vi "SalvaImpostazioniFunzioniCorrettrici_INPUT.vi"(11 "Valore letto da DAQ":dbl) -> ()   [LabVIEW 2019]
uses:
  <vilib>/Utility/miscctls.llb/LVRowAndColumnTypeDef.ctl
  <vilib>/Analysis/6fits.llb/Curve Fitting Criteria.ctl
  <vilib>/Analysis/polynomials.llb/Polynomial Plot (Range).vi
  <vilib>/Analysis/NI_AALPro.lvlib
panel:
  out "Sensore selezionato":string
  in  "Elimina Funzione Correttrice":bool
  out "Ingresso Selezionato":string
  in  "Ordine Polinomio Fit":i32=2
  out "Contenuto file":string[][](array[string])
  out "Indice Sensore":i32
  in  "Tabella Acquisizioni":i32(listbox)
  in  "Valore Letto da sensore":dbl
  in  "Acquisici Punto":bool
  in  "Salva Dati":bool
  in  "Analizza Dati":bool
  in  "Elimina Ultimo Punto":bool
  in  "stop":bool
  out "Graph":cluster{"Ramp Pattern":dbl[], "P(A)":dbl[]}[](graph)
  in  "Stato Sensori":i32(listbox)
  out "transposed array":string[][](array[string])
  out "Array":string[][](array[string])
  out "array w/ subset deleted":string[][](array[string])
  out "output array 2":string[][](array[string])
  out "output array":string[][](array[string])
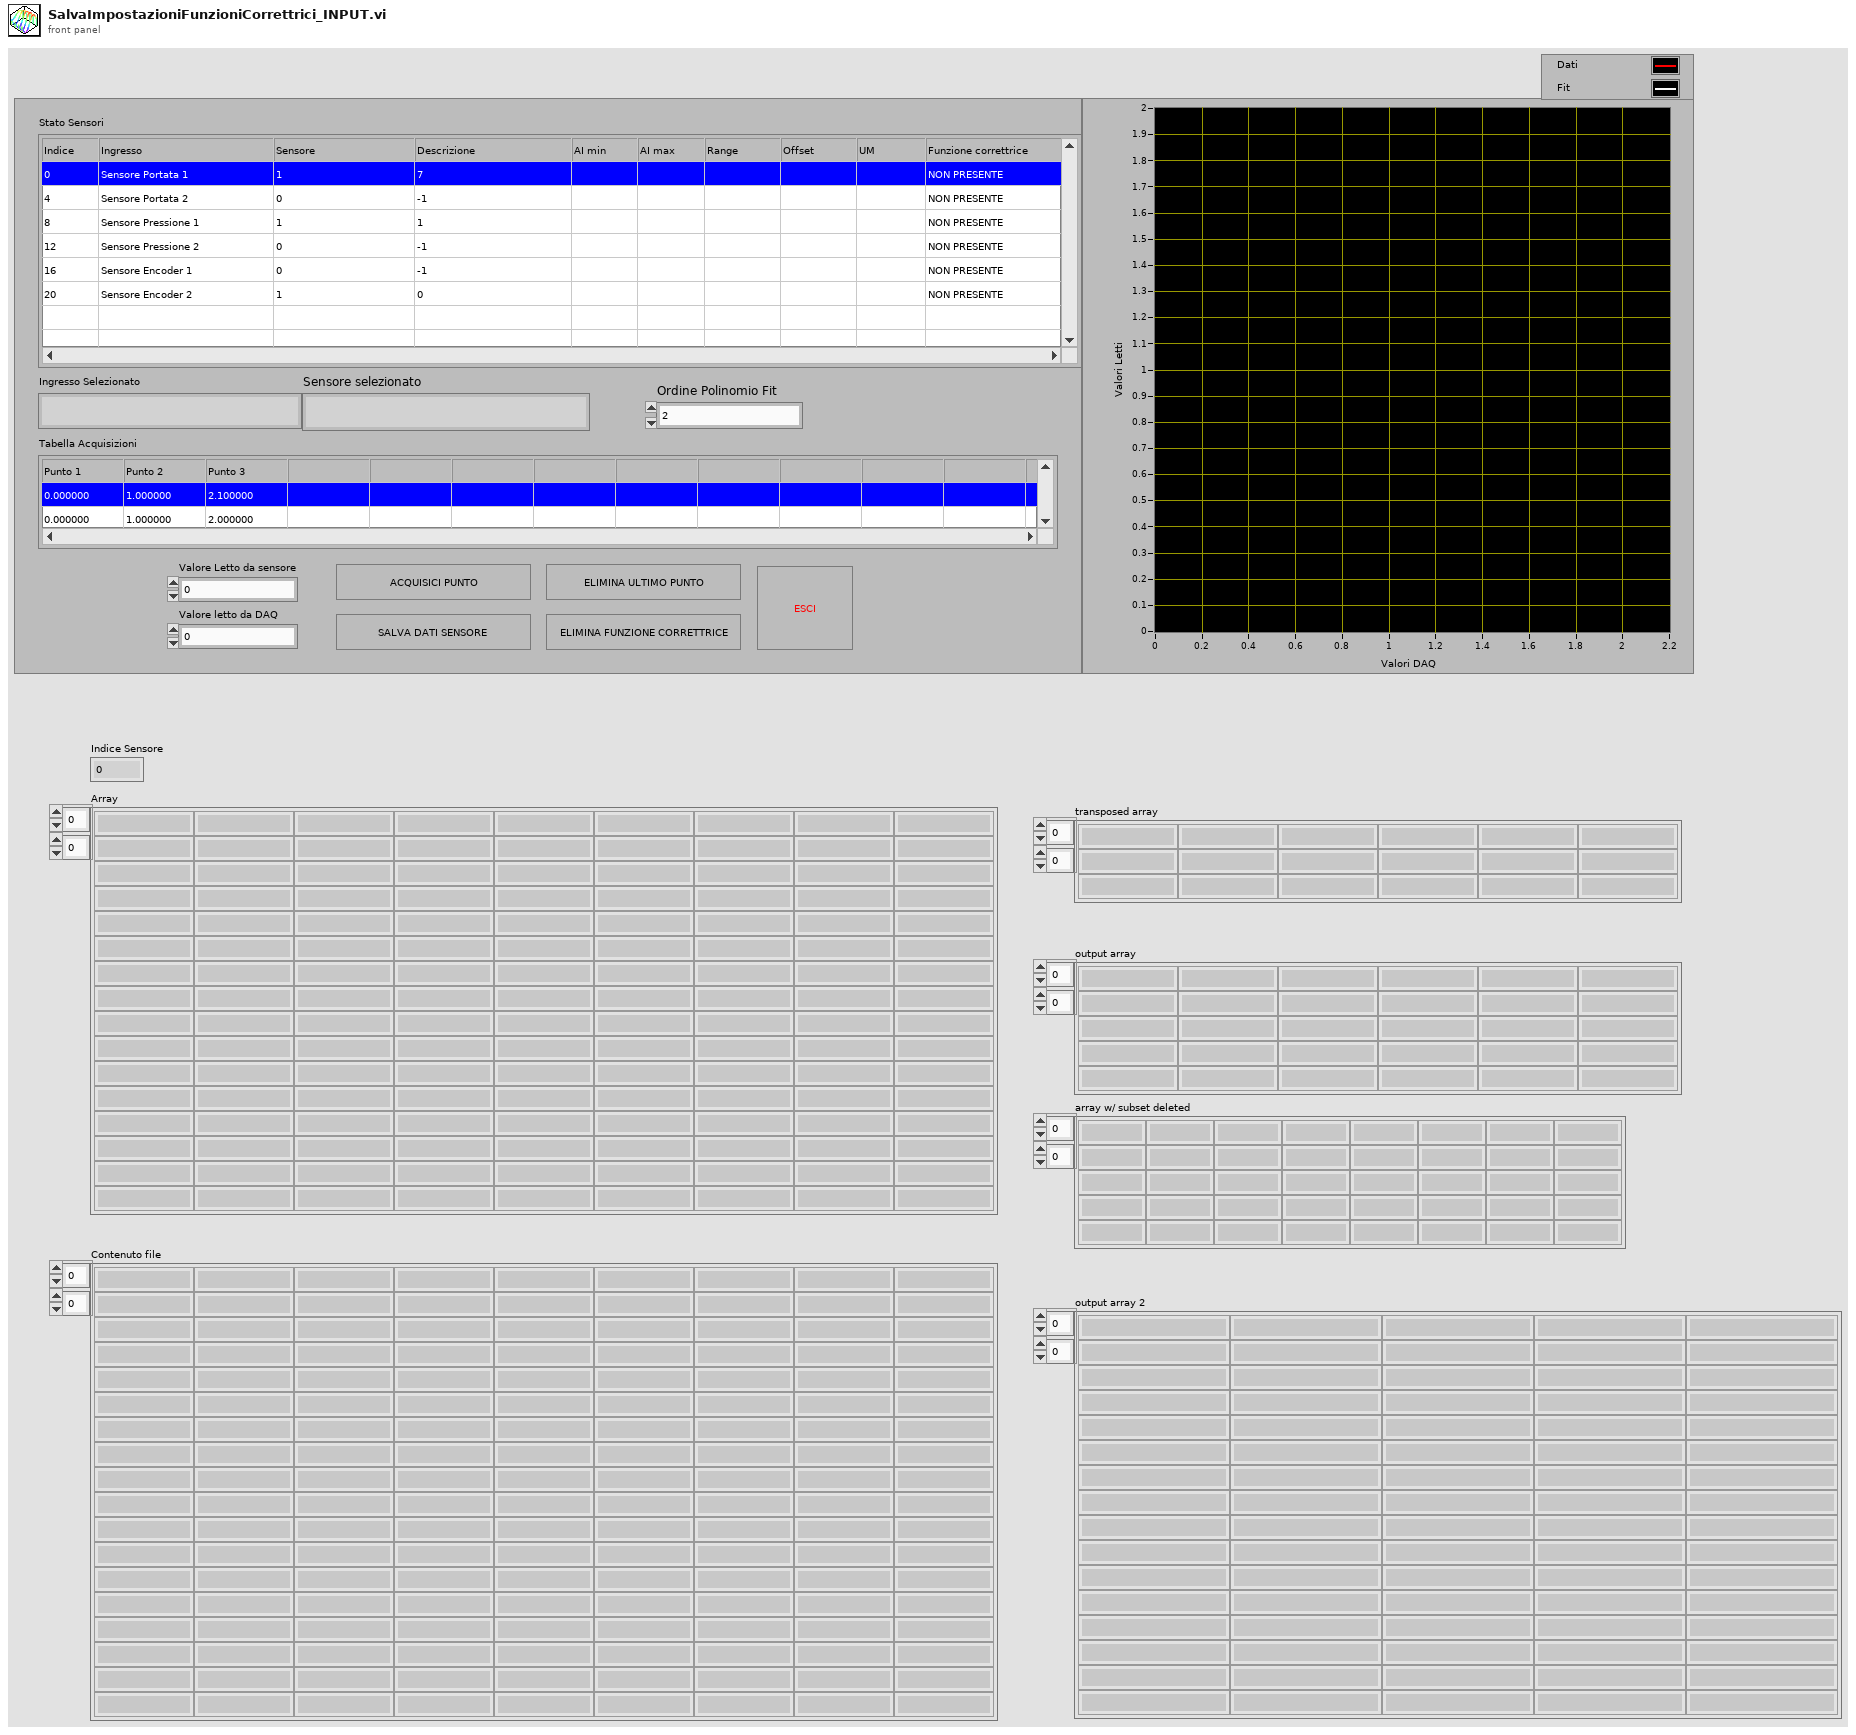
[diagram p1: front panel]
types:
  T1 = typedef "LVRowAndColumnTypeDef.ctl" = cluster{"Row":i32, "Column":i32}
  T2 = enum16{"open", "replace", "create", "open or create", "replace or create", "replace or create with confirmation"}
  T3 = typedef "NI_AALPro.lvlib/Curve Fitting Criteria.ctl" = u16
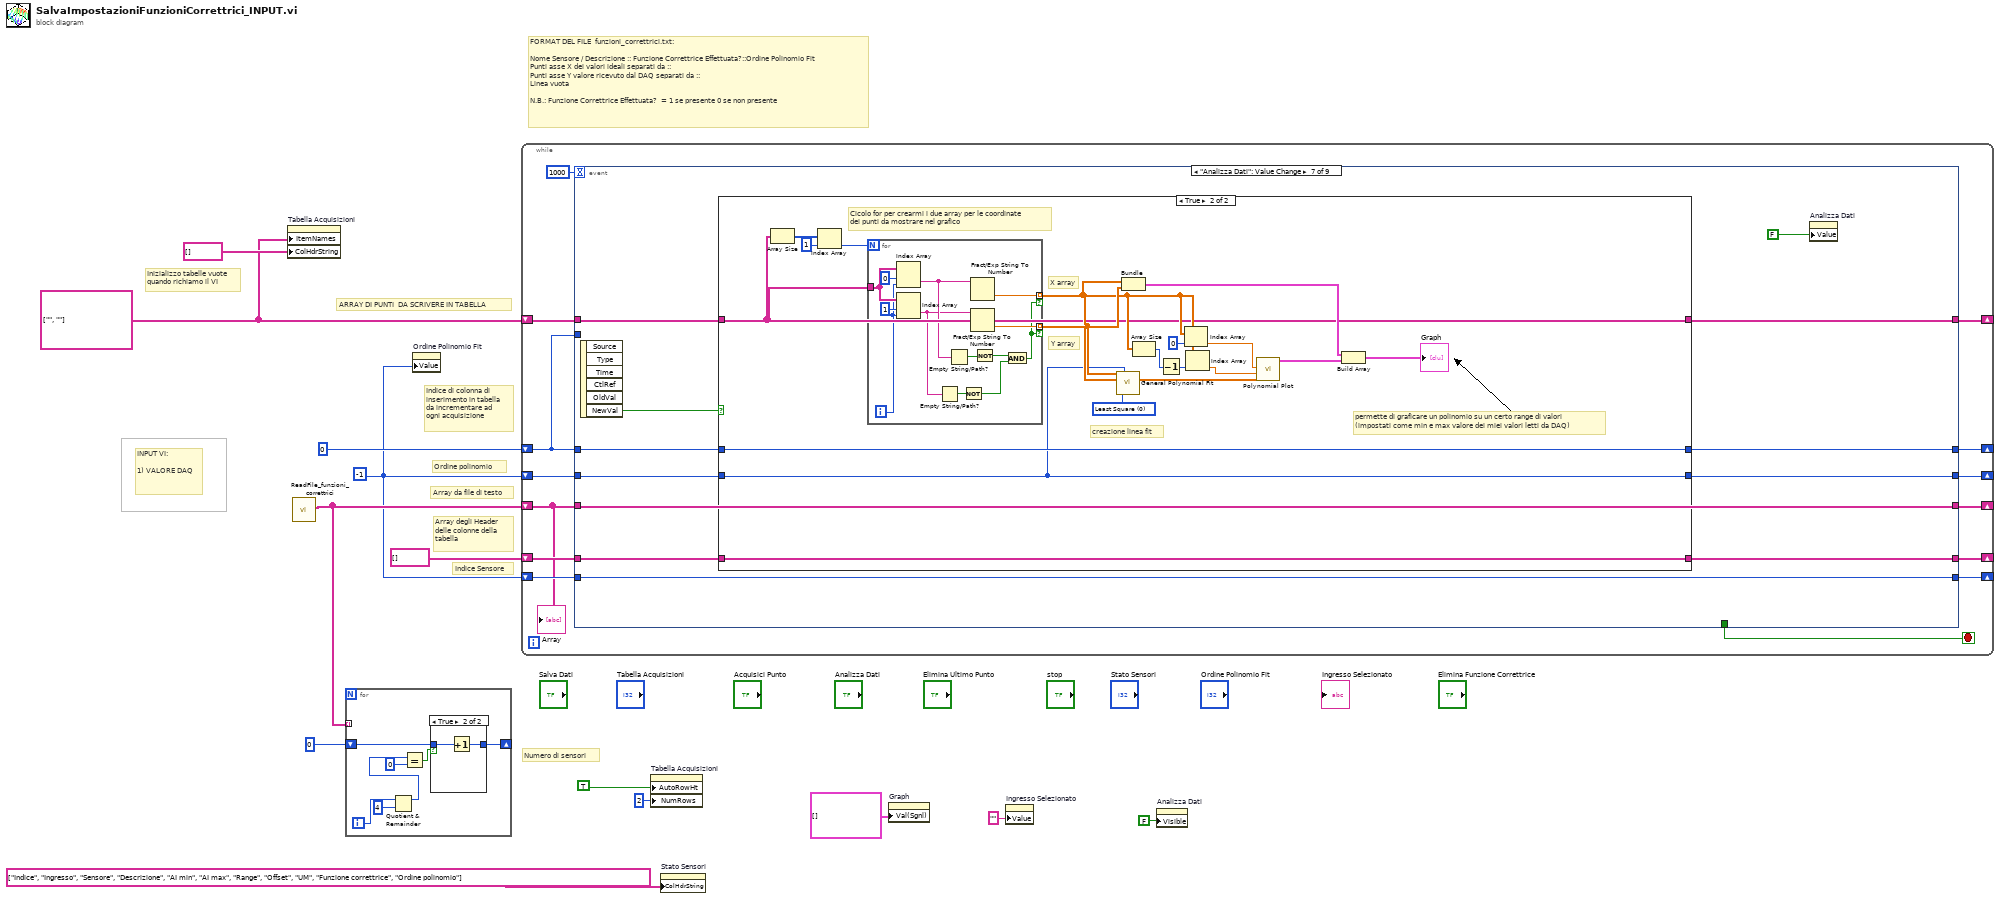
[diagram p0: block diagram]
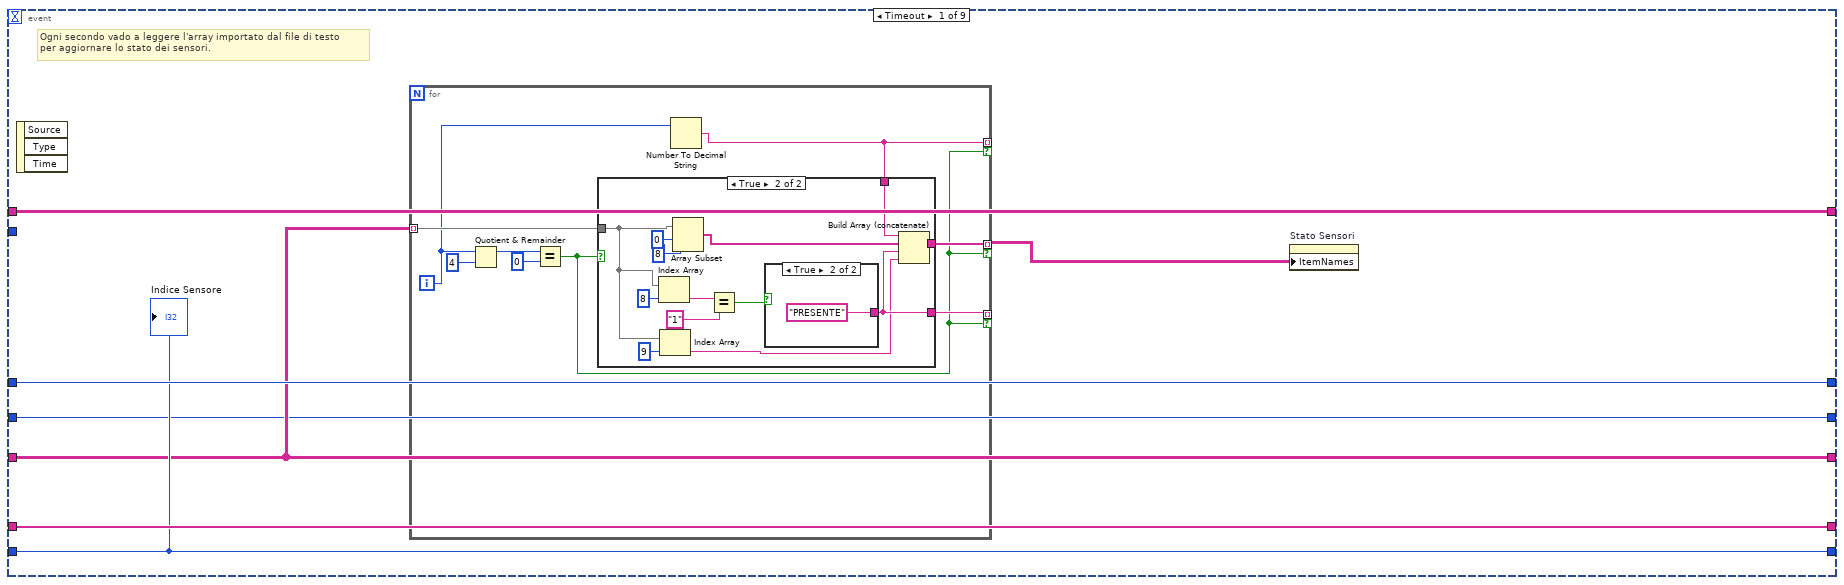
[diagram p3: hidden frame]
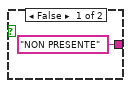
[diagram p5: hidden frame]
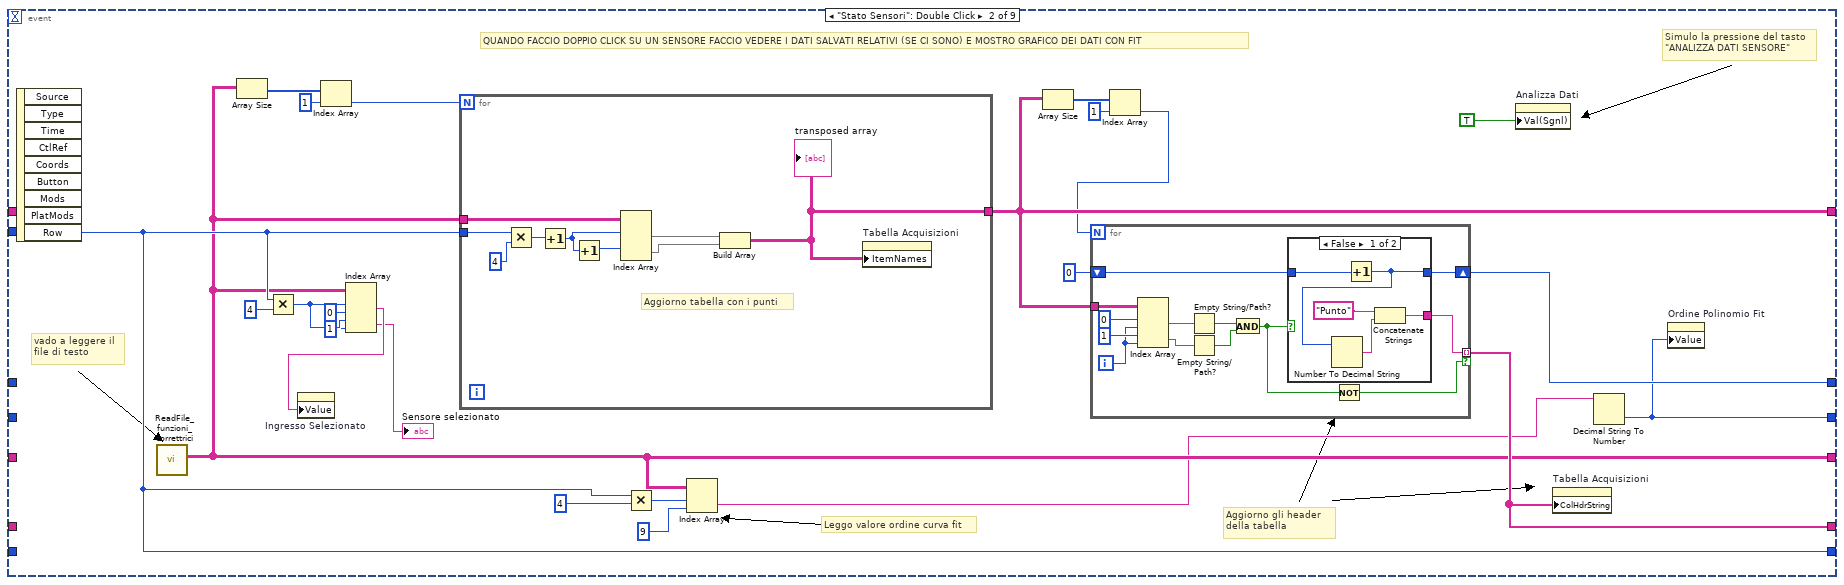
[diagram p6: hidden frame]
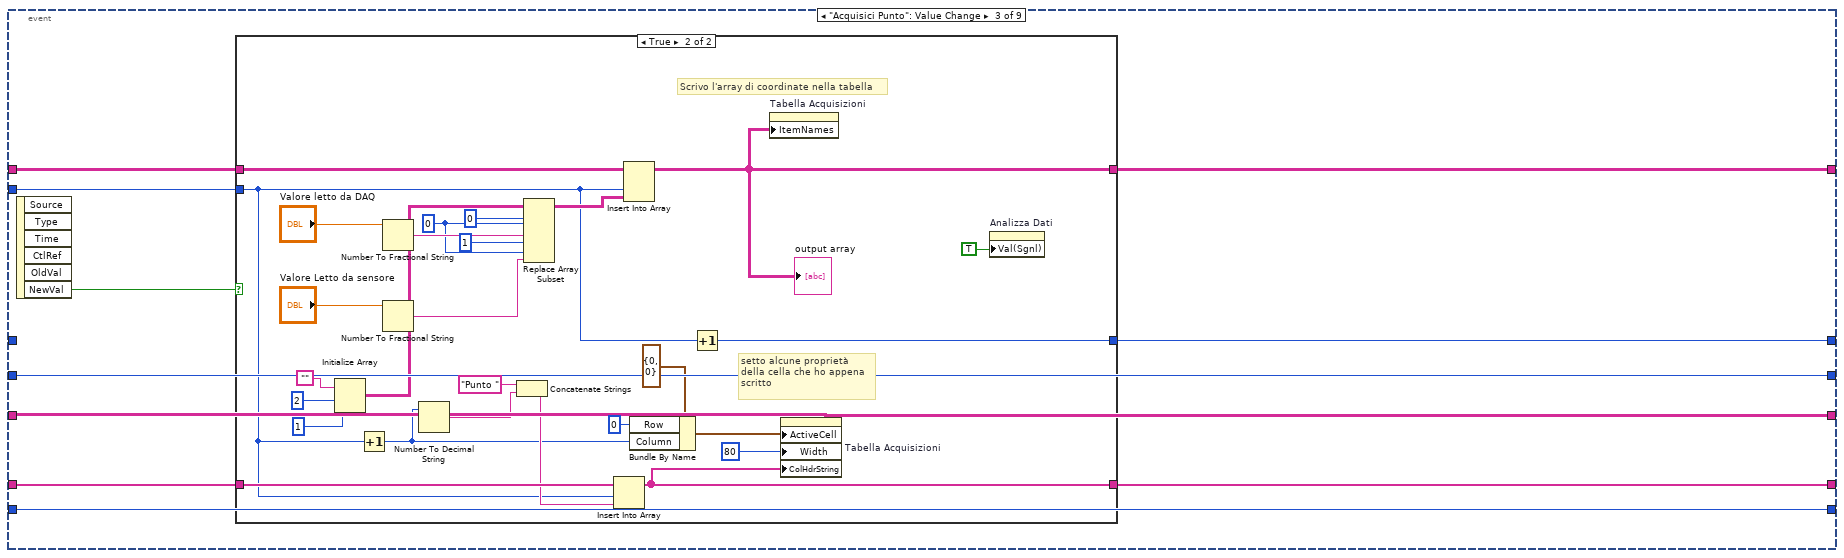
[diagram p8: hidden frame]
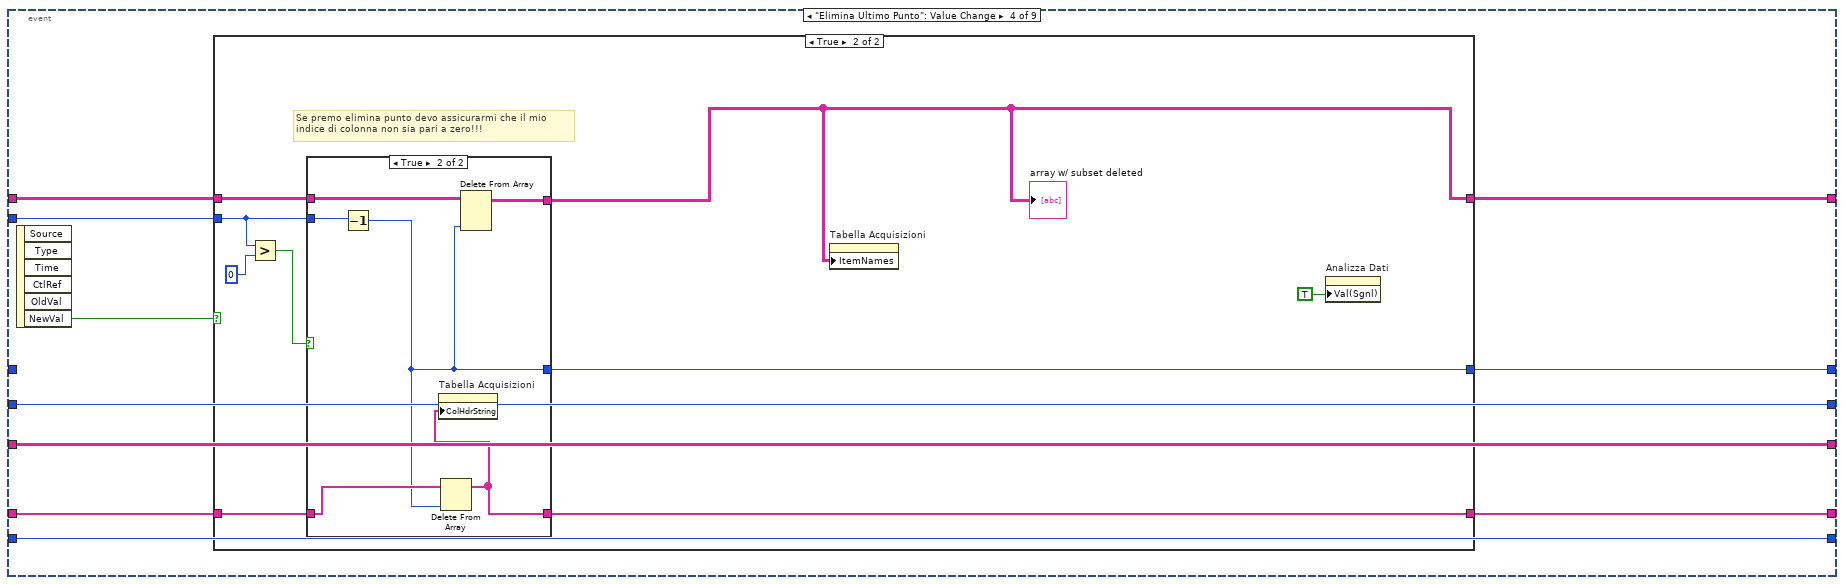
[diagram p10: hidden frame]
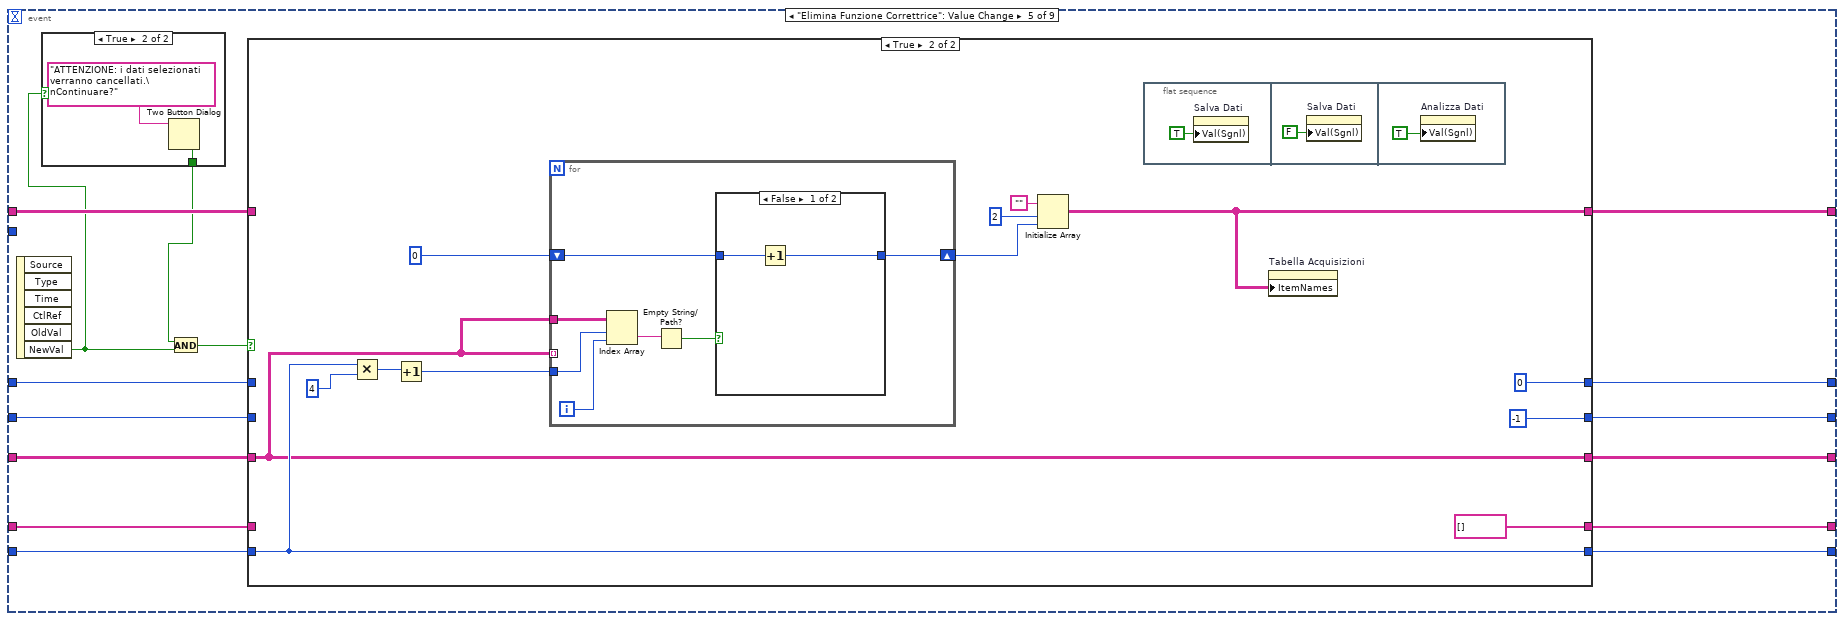
[diagram p13: hidden frame]
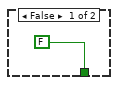
[diagram p14: hidden frame]
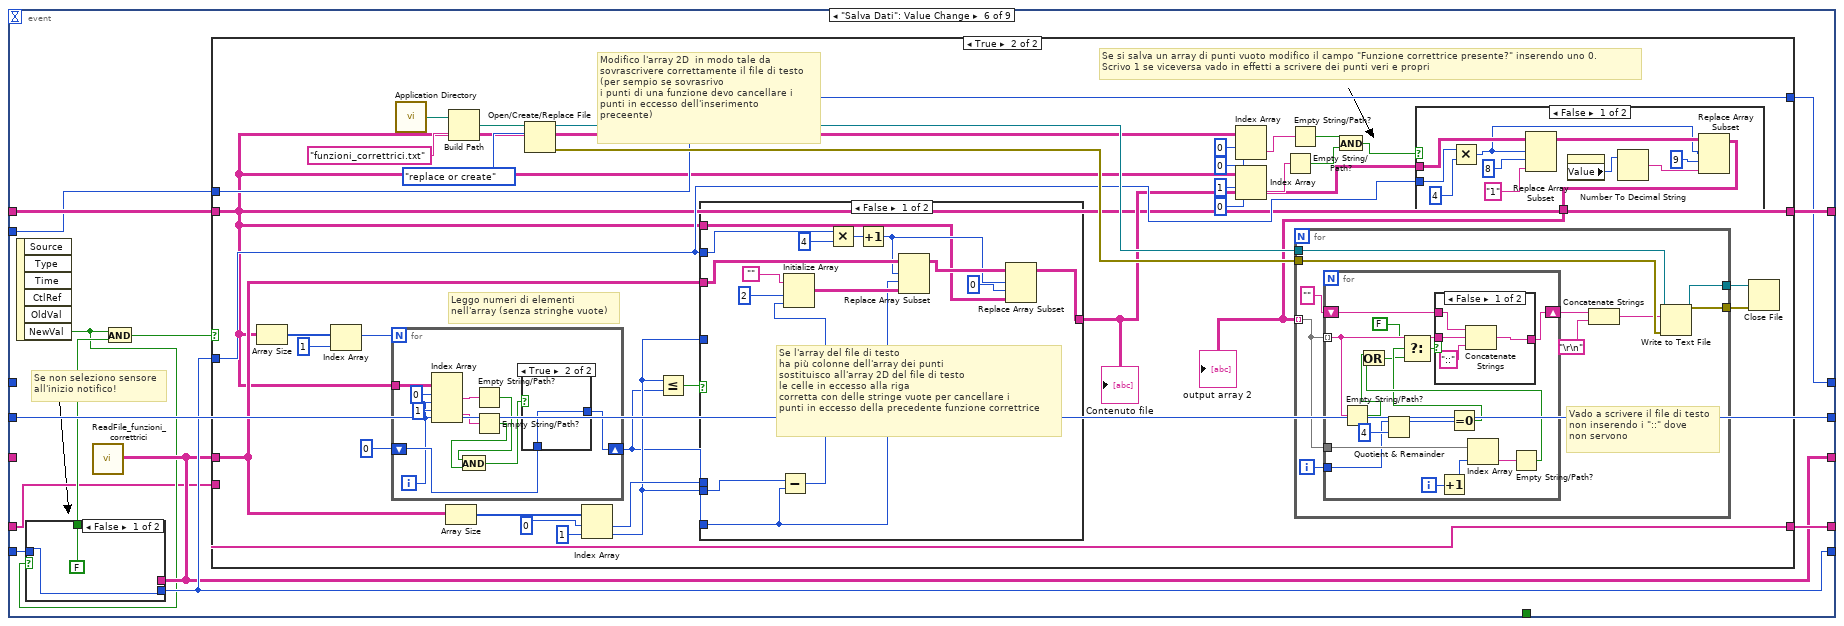
[diagram p17: hidden frame]
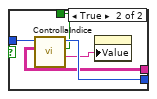
[diagram p18: hidden frame]
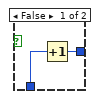
[diagram p20: hidden frame]
diagram:
  w2 = -1 ("Value")
  w6 = string[][] [[""], [""]] ("Item Names")
  # "FORMAT DEL FILE  funzioni_correttrici.txt:\n\nNome Sensore / Descrizione :: Funzione Correttrice Effettuata?::Ordine Polinomio Fit \nPunti asse X dei valori ideali separati da ::\nPunti asse Y valore ricevuto dal DAQ separati da ::\nLinea vuota\n\nN.B.: Funzione Correttrice Effettuata?  = 1 se presente 0 se non presente"
  # "Ordine polinomio"
  # "Numero di sensori"
  # "INPUT VI:\n\n1) VALORE DAQ"
  # "Array da file di testo"
  # "Indice Sensore"
  # "Array degli Header\ndelle colonne della \ntabella"
  # "Indice di colonna di \ninserimento in tabella\nda incrementare ad \nogni acquisizione"
  # "ARRAY DI PUNTI  DA SCRIVERE IN TABELLA"
  # "Inizializzo tabelle vuote\nquando richiamo il VI"
  n1 = property on="Tabella Acquisizioni" class="MCListbox (strict)"("ItemNames"=w6, "ColHdrString"=string[] [] ("Column Header Strings[]")) -> ()  [unwired: 2 in, 2 out]
  n2 = call "ReadFile_funzioni_correttrici.vi"() -> ("Contenuto file"=w4:string[][])  [unwired: 11 in]
  n3 = for {
    tunnel: w4 -> [_] mode=indexing
    shift-right: [w17] -> _
    shift-left: 0 -> [w18]
    i -> [w20]
    n4 = Quotient & Remainder(x=w20, y=4) -> (x-y*floor(x/y)=w16:i32)  [unwired: 1 out]
    n5 = Equal?(x=w16, y=0) -> (x = y?=w14:bool)
    n6 = case shown="True" w14 {
      tunnel: w18 -> [w21 w23]
      tunnel: [w21 w22] -> w17
      frame False {
      }
      frame True {
        n7 = Increment(x=w23) -> (x+1=w22:i32)
      }
    }
  }
  n8 = property on="Ordine Polinomio Fit" class="DigNum (strict)"("Value"=w2) -> ()  [unwired: 2 in, 2 out]
  n9 = while {
    shift-right: [w36] -> _
    shift-left: 0 -> [w30]
    shift-right: [w35] -> _
    shift-left: w6 -> [w37]
    shift-right: [w33] -> _
    shift-left: string[] [] ("Column Header Strings[]") -> [w34]
    shift-right: [w29] -> _
    shift-left: w4 -> [w26]
    shift-right: [w27] -> _
    shift-left: w2 -> [w32]
    shift-right: [w25] -> _
    shift-left: w2 -> [w24]
    stop <- w31 stop-if-true
    n10 = event shown="[6] \"Analizza Dati\": Value Change" {
      selector: _ -> [_ _ _ _ _ _ _ _ _]
      dyn-events: _ -> [_ _ _ _ _ _ _ _ _]
      timeout: 1000 -> [_ _ _ _ _ _ _ _ _]
      tunnel: w37 -> [w44 _ w129 w169 w202 w253 w410 w454 _]
      tunnel: w30 -> [_ _ w128 w168 _ w250 _ _ _]
      tunnel: [w43 w84 w127 w166 w198 w251 w409 w450 _] -> w36
      tunnel: [w44 w89 w126 w167 w201 w252 w411 w454 _] -> w35
      tunnel: w34 -> [w42 _ w125 w164 w195 w242 w407 w453 _]
      tunnel: [w42 w83 w124 w165 w196 w254 w406 w453 _] -> w33
      tunnel: w26 -> [w40 _ w123 w163 w205 _ w405 w452 _]
      tunnel: w32 -> [w41 _ w122 w162 w204 w248 w404 w451 _]
      tunnel: [_ _ _ _ _ _ _ _ TRUE] -> w31
      tunnel: w30 -> [w43 _ _ _ w197 _ w408 w450 _]
      tunnel: [w40 w73 w123 w163 w206 w244 w405 w452 _] -> w29
      tunnel: [w41 w74 w122 w162 w203 w247 w404 w451 _] -> w27
      tunnel: [w39 w78 w121 w161 w199 w249 w402 w449 _] -> w25
      tunnel: w24 -> [w39 _ w121 w161 w200 w249 w401 _ _]
      event Timeout {
        # "Ogni secondo vado a leggere l'array importato dal file di testo \nper aggiornare lo stato dei sensori."
        n11 = event-data() -> ()  [unwired: 1 in, 3 out]
        n12 = for {
          tunnel: w40 -> [w50] mode=indexing
          tunnel: [w49] -> _ mode=indexing if=w47
          tunnel: [w48] -> w38 mode=indexing if=w47
          tunnel: [w45] -> _ mode=indexing if=w47
          i -> [w46]
          n13 = Quotient & Remainder(x=w46, y=4) -> (x-y*floor(x/y)=w52:i32)  [unwired: 1 out]
          n14 = Equal?(x=w52, y=0) -> (x = y?=w47:bool)
          n15 = Number To Decimal String(number=w46) -> (decimal integer string=w45:string)  [unwired: 1 in]
          n16 = case shown="True" w47 {
            tunnel: w50 -> [_ w56]
            tunnel: [_ w59] -> w48
            tunnel: [_ w57] -> w49
            tunnel: w45 -> [_ w58]
            frame False {
            }
            frame True {
              n17 = Index Array(array=w56, index=8) -> (element=w65:string)
              n18 = Index Array(array=w56, index=9) -> (element=w54:string)
              n19 = Array Subset(array=w56, index=0, length=8) -> (w62:string[])
              n20 = Equal?(x=w65, y="1") -> (x = y?=w63:bool)
              n21 = case shown="True" w63 {
                tunnel: ["NON PRESENTE" "PRESENTE"] -> w57
                frame False {
                }
                frame True {
                }
              }
              n22 = Build Array (concatenate)(w58, w62, w57, w54) -> (w59:string[])
            }
          }
        }
        n23 = property on="Stato Sensori" class="MCListbox (strict)"("ItemNames"=w38) -> ()  [unwired: 2 in, 2 out]
        "Indice Sensore" <- w41
      }
      event "Stato Sensori": Double Click {
        # "Leggo valore ordine curva fit"
        # "Aggiorno gli header \ndella tabella"
        # "Simulo la pressione del tasto\n\"ANALIZZA DATI SENSORE\""
        # "QUANDO FACCIO DOPPIO CLICK SU UN SENSORE FACCIO VEDERE I DATI SALVATI RELATIVI (SE CI SONO) E MOSTRO GRAFICO DEI DATI CON FIT"
        # "vado a leggere il \nfile di testo"
        n24 = event-data() -> ("Row"=w74:i32)  [unwired: 1 in, 8 out]
        n25 = call "ReadFile_funzioni_correttrici.vi"() -> ("Contenuto file"=w73:string[][])  [unwired: 11 in]
        n26 = Array Size(array=w73) -> (size(s)=w91:i32[])
        n27 = Multiply(x=w74, y=4) -> (x*y=w72:i32)
        n28 = Index Array(array=w91, index=1) -> (element=w92:i32)
        n29 = Index Array(array=w73, index (row) #1=w72, index (col) #1=0 ("disabled index (col)"), index (row) #2=w72, index (col) #2=1 ("disabled index (col)")) -> (element #1=w76:string, element #2=→"Sensore selezionato":string)
        n30 = property on="Ingresso Selezionato" class="Str"("Value"=w76) -> ()  [unwired: 2 in, 2 out]
        n31 = for {
          N: w92 -> [_]
          tunnel: w73 -> [w120]
          tunnel: w74 -> [w119]
          tunnel: [w112] -> w89
          # "Aggiorno tabella con i punti"
          n32 = Multiply(x=w119, y=4) -> (x*y=w117:i32)
          n33 = Increment(x=w117) -> (x+1=w115:i32)
          n34 = Increment(x=w115) -> (x+1=w116:i32)
          n35 = Index Array(array=w120, index (row) #1=w115, index (row) #2=w116) -> (element #1=w114:string[], element #2=w113:string[])  [unwired: 2 in]
          n36 = Build Array(w114, w113) -> (w112:string[][])
          "transposed array" <- w112
          n37 = property on="Tabella Acquisizioni" class="MCListbox (strict)"("ItemNames"=w112) -> ()  [unwired: 2 in, 2 out]
        }
        n38 = Multiply(x=w74, y=4) -> (x*y=w81:i32)
        n39 = Index Array(array=w73, index (row)=w81, index (col)=9 ("disabled index (col)")) -> (element=w69:string)
        n40 = Array Size(array=w89) -> (size(s)=w88:i32[])
        n41 = Index Array(array=w88, index=1) -> (element=w86:i32)
        n42 = for {
          N: w86 -> [_]
          tunnel: w89 -> [w105]
          shift-right: [w96] -> w84
          shift-left: 0 -> [w97]
          tunnel: [w95] -> w83 mode=indexing if=w93
          i -> [w102]
          n43 = Index Array(array=w105, index (row) #1=0 ("index (row)"), index (col) #1=w102, index (row) #2=1 ("index (row)"), index (col) #2=w102) -> (element #1=w101:string, element #2=w100:string)
          n44 = Empty String/Path?(string/path=w101) -> (empty?=w99:bool)
          n45 = Empty String/Path?(string/path=w100) -> (empty?=w98:bool)
          n46 = And(x=w99, y=w98) -> (x .and. y?=w94:bool)
          n47 = case shown="False" w94 {
            tunnel: w97 -> [w110 w111]
            tunnel: [w108 w111] -> w96
            tunnel: [w106 _] -> w95
            frame False {
              n48 = Increment(x=w110) -> (x+1=w108:i32)
              n49 = Number To Decimal String(number=w108) -> (decimal integer string=w107:string)  [unwired: 1 in]
              n50 = Concatenate Strings("Punto", w107) -> (w106:string)
            }
            frame True {
            }
          }
          n51 = Not(x=w94) -> (.not. x?=w93:bool)
        }
        n52 = property on="Analizza Dati" class="Bool (strict)"("Val(Sgnl)"=TRUE ("Value (Signaling)")) -> ()  [unwired: 2 in, 2 out]
        n53 = property on="Tabella Acquisizioni" class="MCListbox (strict)"("ColHdrString"=w83) -> ()  [unwired: 2 in, 2 out]
        n54 = Decimal String To Number(string=w69) -> (number=w78:i32)  [unwired: 2 in, 1 out]
        n55 = property on="Ordine Polinomio Fit" class="DigNum (strict)"("Value"=w78) -> ()  [unwired: 2 in, 2 out]
      }
      event "Acquisici Punto": Value Change {
        n56 = event-data() -> ("NewVal"=w130:bool)  [unwired: 1 in, 5 out]
        n57 = case shown="True" w130 {
          tunnel: w129 -> [w132 w149]
          tunnel: w128 -> [w133 w136]
          tunnel: [w133 w147] -> w127
          tunnel: [w132 w146] -> w126
          tunnel: w125 -> [w131 w141]
          tunnel: [w131 w137] -> w124
          frame False {
          }
          frame True {
            w152 = 0 ("disabled index (col)")
            # "setto alcune proprietà \ndella cella che ho appena\nscritto"
            # "Scrivo l'array di coordinate nella tabella"
            n58 = Initialize Array("", 2 ("dimension size"), 1 ("dimension size")) -> (w155:string[][])
            n59 = Increment(x=w136) -> (x+1=w135:i32)
            n60 = Number To Fractional String(number="Valore letto da DAQ") -> (F-format string=w154:string)  [unwired: 3 in]
            n61 = Number To Fractional String(number="Valore Letto da sensore") -> (F-format string=w150:string)  [unwired: 3 in]
            n62 = Number To Decimal String(number=w135) -> (decimal integer string=w138:string)  [unwired: 1 in]
            n63 = Concatenate Strings("Punto ", w138) -> (w139:string)
            n64 = Replace Array Subset(array=w155, new element #1=w154, index (row) #1=0 ("index (row)"), index (col) #1=w152, new element #2=w150, index (row) #2=1 ("disabled index (row)"), index (col) #2=w152) -> (w148:string[][])
            n65 = Insert Into Array(array=w141, index=w136, new element=w139) -> (w137:string[])
            n66 = Insert Into Array(array=w149, index (col)=w136, new element=w148) -> (w146:string[][])  [unwired: 1 in]
            "output array" <- w146
            n67 = Bundle By Name(cluster=T1 {"Row"=0, "Column"=0} ("Active Cell:Active Cell"), "Row"=0, "Column"=w135) -> (w144:T1)
            n68 = Increment(x=w136) -> (x+1=w147:i32)
            n69 = property on="Tabella Acquisizioni" class="MCListbox (strict)"("ItemNames"=w146) -> ()  [unwired: 2 in, 2 out]
            n70 = property on="Tabella Acquisizioni" class="MCListbox (strict)"("ActiveCell"=w144, "Width"=u32 80 ("Active Cell:Cell Size:Width"), "ColHdrString"=w137) -> ()  [unwired: 2 in, 2 out]
            n71 = property on="Analizza Dati" class="Bool (strict)"("Val(Sgnl)"=TRUE ("Analizza Dati")) -> ()  [unwired: 2 in, 2 out]
          }
        }
      }
      event "Elimina Ultimo Punto": Value Change {
        n72 = event-data() -> ("NewVal"=w170:bool)  [unwired: 1 in, 5 out]
        n73 = case shown="True" w170 {
          tunnel: w169 -> [w173 w176]
          tunnel: w168 -> [w172 w180]
          tunnel: [w173 w175] -> w167
          tunnel: [w172 w181] -> w166
          tunnel: [w171 w177] -> w165
          tunnel: w164 -> [w171 w182]
          frame False {
          }
          frame True {
            # "Se premo elimina punto devo assicurarmi che il mio \nindice di colonna non sia pari a zero!!!"
            n74 = Greater?(x=w180, y=0) -> (0:w178:bool)
            n75 = case shown="True" w178 {
              tunnel: w182 -> [w184 w191]
              tunnel: [w185 w187] -> w181
              tunnel: w180 -> [w185 w190]
              tunnel: [w184 w189] -> w177
              tunnel: w176 -> [w183 w188]
              tunnel: [w183 w186] -> w175
              frame False {
              }
              frame True {
                n76 = Decrement(x=w190) -> (x-1=w187:i32)
                n77 = Delete From Array(array=w191, index=w187) -> (array with subset deleted=w189:string[])  [unwired: 1 in, 1 out]
                n78 = property on="Tabella Acquisizioni" class="MCListbox (strict)"("ColHdrString"=w189) -> ()  [unwired: 2 in, 2 out]
                n79 = Delete From Array(array=w188, index (col)=w187) -> (array with subset deleted=w186:string[][])  [unwired: 2 in, 1 out]
              }
            }
            "array w/ subset deleted" <- w175
            n80 = property on="Tabella Acquisizioni" class="MCListbox (strict)"("ItemNames"=w175) -> ()  [unwired: 2 in, 2 out]
            n81 = property on="Analizza Dati" class="Bool (strict)"("Val(Sgnl)"=TRUE ("Analizza Dati")) -> ()  [unwired: 2 in, 2 out]
          }
        }
      }
      event "Elimina Funzione Correttrice": Value Change {
        n82 = event-data() -> ("NewVal"=w194:bool)  [unwired: 1 in, 5 out]
        n83 = case shown="True" w194 {
          tunnel: [FALSE w208] -> w192
          frame False {
          }
          frame True {
            n84 = Two Button Dialog(message="ATTENZIONE: i dati selezionati verranno cancellati.\nContinuare?") -> (T button?=w208:bool)  [unwired: 2 in]
          }
        }
        n85 = And(x=w192, y=w194) -> (x .and. y?=w193:bool)
        n86 = case shown="True" w193 {
          tunnel: [w215 w216] -> w206
          tunnel: w205 -> [w215 w216]
          tunnel: [w214 w228] -> w203
          tunnel: w204 -> [w214 w228]
          tunnel: w202 -> [w213 _]
          tunnel: [w213 w217] -> w201
          tunnel: w200 -> [w212 _]
          tunnel: [w212 -1 ("Value")] -> w199
          tunnel: w197 -> [w211 _]
          tunnel: [w211 0] -> w198
          tunnel: [w210 string[] [] ("Column Header Strings[]")] -> w196
          tunnel: w195 -> [w210 _]
          frame False {
          }
          frame True {
            n87 = Multiply(x=w228, y=4 ("Value")) -> (x*y=w226:i32)
            n88 = Increment(x=w226) -> (x+1=w224:i32)
            n89 = for {
              shift-right: [w232] -> w222
              shift-left: 0 ("Value") -> [w233]
              tunnel: w216 -> [_] mode=indexing
              tunnel: w224 -> [w237]
              tunnel: w216 -> [w238]
              i -> [w236]
              n90 = Index Array(array=w238, index (row)=w237, index (col)=w236) -> (element=w235:string)
              n91 = Empty String/Path?(string/path=w235) -> (empty?=w234:bool)
              n92 = case shown="False" w234 {
                tunnel: w233 -> [w240 w241]
                tunnel: [w239 w241] -> w232
                frame False {
                  n93 = Increment(x=w240) -> (x+1=w239:i32)
                }
                frame True {
                }
              }
            }
            n94 = Initialize Array("", 2 ("dimension size"), w222) -> (w217:string[][])
            n95 = flat-sequence {
              frame #0 {
                n96 = property on="Salva Dati" class="Bool (strict)"("Val(Sgnl)"=TRUE ("Value (Signaling)")) -> ()  [unwired: 2 in, 2 out]
              }
              frame #1 {
                n97 = property on="Salva Dati" class="Bool (strict)"("Val(Sgnl)"=FALSE ("Value (Signaling)")) -> ()  [unwired: 2 in, 2 out]
              }
              frame #2 {
                n98 = property on="Analizza Dati" class="Bool (strict)"("Val(Sgnl)"=TRUE ("Analizza Dati")) -> ()  [unwired: 2 in, 2 out]
              }
            }
            n99 = property on="Tabella Acquisizioni" class="MCListbox (strict)"("ItemNames"=w217) -> ()  [unwired: 2 in, 2 out]
          }
        }
      }
      event "Salva Dati": Value Change {
        # "Se non seleziono sensore\nall'inizio notifico!"
        n100 = event-data() -> ("NewVal"=w243:bool)  [unwired: 1 in, 5 out]
        n101 = call "ReadFile_funzioni_correttrici.vi"() -> ("Contenuto file"=w244:string[][])  [unwired: 11 in]
        n102 = case shown="False" w243 {
          tunnel: w248 -> [w255 w261]
          tunnel: [w255 w260] -> w247
          tunnel: [FALSE ("OK") w259] -> w245
          tunnel: w244 -> [_ w258]
          frame False {
          }
          frame True {
            n103 = call "ControllaIndice.vi"("Contenuto file 2"=w258, "Indice Sensore"=w261) -> ("Sensore Selez."=w257:string, "OK"=w259:bool, "Indice Sensore 2"=w260:i32)  [unwired: 7 in]
            n104 = property on="Ingresso Selezionato" class="Str"("Value"=w257) -> ()  [unwired: 2 in, 2 out]
          }
        }
        n105 = And(x=w243, y=w245) -> (x .and. y?=w246:bool)
        n106 = case shown="True" w246 {
          tunnel: w244 -> [_ w292]
          tunnel: w247 -> [_ w272]
          tunnel: w242 -> [w264 w288]
          tunnel: [w264 w288] -> w254
          tunnel: w253 -> [w263 w265]
          tunnel: [w263 w265] -> w252
          tunnel: [w262 w266] -> w251
          tunnel: w250 -> [w262 w266]
          frame False {
          }
          frame True {
            # "Leggo numeri di elementi\nnell'array (senza stringhe vuote)"
            # "Se si salva un array di punti vuoto modifico il campo \"Funzione correttrice presente?\" inserendo uno 0.\nScrivo 1 se viceversa vado in effetti a scrivere dei punti veri e propri"
            # "Modifico l'array 2D  in modo tale da \nsovrascrivere correttamente il file di testo \n(per sempio se sovrasrivo\ni punti di una funzione devo cancellare i \npunti in eccesso dell'inserimento \npreceente)"
            n107 = Array Size(array=w265) -> (size(s)=w299:i32[])
            n108 = Index Array(array=w299, index=1) -> (element=w268:i32)
            n109 = for {
              N: w268 -> [_]
              tunnel: w265 -> [w310]
              shift-right: [w301] -> w267
              shift-left: 0 -> [w302]
              i -> [w300]
              n110 = Index Array(array=w310, index (row) #1=0 ("disabled index (row)"), index (col) #1=w300, index (row) #2=1 ("disabled index (row)"), index (col) #2=w300) -> (element #1=w307:string, element #2=w306:string)
              n111 = Empty String/Path?(string/path=w307) -> (empty?=w305:bool)
              n112 = Empty String/Path?(string/path=w306) -> (empty?=w304:bool)
              n113 = And(x=w305, y=w304) -> (x .and. y?=w303:bool)
              n114 = case shown="True" w303 {
                tunnel: w302 -> [w312 w313]
                tunnel: [w311 w313] -> w301
                frame False {
                  n115 = Increment(x=w312) -> (x+1=w311:i32)
                }
                frame True {
                }
              }
            }
            n116 = call <vilib>:"Application Directory.vi"() -> ("Application Directory"=w284:path)
            n117 = Array Size(array=w292) -> (size(s)=w297:i32[])
            n118 = Build Path(base path=w284, name or relative path="funzioni_correttrici.txt") -> (appended path=w283:path)
            n119 = Open/Create/Replace File(file path (use dialog)=w283, operation (0:open)=T2."replace or create") -> (refnum out=w286:refnum<file>, error out=w285:errorcluster)  [unwired: 4 in, 1 out]
            n120 = Index Array(array=w297, index #1=0 ("index"), index #2=1 ("index")) -> (element #1=w294:i32, element #2=w291:i32)
            n121 = Less Or Equal?(x=w291, y=w267) -> (x <= y?=w293:bool)
            n122 = case shown="False" w293 {
              tunnel: w294 -> [_ w400]
              tunnel: w291 -> [w383 w397]
              tunnel: w267 -> [w369 w384]
              tunnel: w292 -> [w380 w395]
              tunnel: w291 -> [_ w394]
              tunnel: w272 -> [w377 w389]
              tunnel: w265 -> [w372 w387]
              tunnel: [w371 w386] -> w271
              frame False {
                # "Se l'array del file di testo\nha più colonne dell'array dei punti\nsostituisco all'array 2D del file di testo\nle celle in eccesso alla riga \ncorretta con delle stringe vuote per cancellare i  \npunti in eccesso della precedente funzione correttrice"
                n123 = Subtract(x=w383, y=w369) -> (x-y=w381:i32)
                n124 = Initialize Array("", 2 ("dimension size"), w381) -> (w376:string[][])
                n125 = Multiply(x=w377, y=4) -> (x*y=w379:i32)
                n126 = Increment(x=w379) -> (x+1=w373:i32)
                n127 = Replace Array Subset(array=w380, new element=w376, index (row)=w373, index (col)=w369) -> (w375:string[][])
                n128 = Replace Array Subset(array=w375, new element=w372, index (row)=w373, index (col)=0 ("disabled index (col)")) -> (w371:string[][])
              }
              frame True {
                # "Se l'array del file di testo\nha meno colonne dell'array dei punti\naggiungo all'array 2D del file di testo le colonne\nmancanti per una corretta scrittura"
                n129 = Subtract(x=w397, y=w384) -> (x-y=w399:i32)
                n130 = Absolute Value(x=w399) -> (abs(x)=w398:i32)
                n131 = Initialize Array("", w400, w398) -> (w396:string[][])
                n132 = Multiply(x=w389, y=4) -> (x*y=w391:i32)
                n133 = Insert Into Array(array=w395, index (col)=w394, new element=w396) -> (w392:string[][])  [unwired: 1 in]
                n134 = Increment(x=w391) -> (x+1=w388:i32)
                n135 = Replace Array Subset(array=w392, new element=w387, index (row)=w388, index (col)=0 ("disabled index (col)")) -> (w386:string[][])
              }
            }
            "Contenuto file" <- w271
            n136 = Index Array(array=w265, index (row)=0, index (col)=0 ("disabled index (col)")) -> (element=w277:string)
            n137 = Index Array(array=w265, index (row)=1, index (col)=0 ("disabled index (col)")) -> (element=w276:string)
            n138 = Empty String/Path?(string/path=w276) -> (empty?=w274:bool)
            n139 = Empty String/Path?(string/path=w277) -> (empty?=w275:bool)
            n140 = And(x=w275, y=w274) -> (x .and. y?=w273:bool)
            n141 = case shown="False" w273 {
              tunnel: w271 -> [w324 w332]
              tunnel: w272 -> [w323 w331]
              tunnel: [w317 w329] -> w270
              frame False {
                n142 = Multiply(x=w323, y=4) -> (x*y=w315:i32)
                n143 = Replace Array Subset(array=w324, new element="1" ("new element/subarray"), index (row)=w315, index (col)=8 ("disabled index (col)")) -> (w316:string[][])
                n144 = property on="Ordine Polinomio Fit" class="DigNum (strict)"() -> ("Value"=w319:i32)  [unwired: 2 in, 2 out]
                n145 = Number To Decimal String(number=w319) -> (decimal integer string=w318:string)  [unwired: 1 in]
                n146 = Replace Array Subset(array=w316, new element=w318, index (row)=w315, index (col)=9 ("disabled index (col)")) -> (w317:string[][])
              }
              frame True {
                w325 = -1 ("number")
                n147 = Multiply(x=w331, y=4) -> (x*y=w328:i32)
                n148 = Replace Array Subset(array=w332, new element="0" ("new element/subarray"), index (row)=w328, index (col)=8 ("disabled index (col)")) -> (w330:string[][])
                n149 = Number To Decimal String(number=w325) -> (decimal integer string=w326:string)  [unwired: 1 in]
                n150 = Replace Array Subset(array=w330, new element=w326, index (row)=w328, index (col)=9 ("disabled index (col)")) -> (w329:string[][])
                n151 = property on="Ordine Polinomio Fit" class="DigNum (strict)"("Value"=w325) -> ()  [unwired: 2 in, 2 out]
              }
            }
            "output array 2" <- w270
            n152 = for {
              tunnel: w270 -> [w343] mode=indexing
              tunnel: [w345] -> w290
              tunnel: [w344] -> w289
              tunnel: w286 -> [w342]
              tunnel: w285 -> [w341]
              i -> [w336]
              # "Vado a scrivere il file di testo\nnon inserendo i \"::\" dove \nnon servono"
              n153 = for {
                tunnel: w343 -> [w354] mode=indexing
                tunnel: w343 -> [w360]
                shift-right: [w361] -> w339
                shift-left: "" -> [w356]
                tunnel: w336 -> [w347]
                i -> [w359]
                n154 = Empty String/Path?(string/path=w354) -> (empty?=w353:bool)
                n155 = Quotient & Remainder(x=w347, y=4) -> (x-y*floor(x/y)=w346:i32)  [unwired: 1 out]
                n156 = Increment(x=w359) -> (x+1=w358:i32)
                n157 = Equal To 0?(x=w346) -> (x = 0?=w351:bool)
                n158 = Index Array(array=w360, index=w358) -> (element=w357:string)
                n159 = Empty String/Path?(string/path=w357) -> (empty?=w355:bool)
                n160 = Or(x=w353, y=w355) -> (x .or. y?=w348:bool)
                n161 = Select(t=FALSE ("f"), s=w351, f=w348) -> (s? t:f=w350:bool)
                n162 = case shown="False" w350 {
                  tunnel: [w364 w366] -> w361
                  tunnel: w354 -> [w363 w367]
                  tunnel: w356 -> [w362 w368]
                  frame False {
                    n163 = Concatenate Strings(w362, w363, "::" ("string")) -> (w364:string)
                  }
                  frame True {
                    n164 = Concatenate Strings(w368, w367) -> (w366:string)
                  }
                }
              }
              n165 = Concatenate Strings(w339, "\r\n") -> (w337:string)
              n166 = Write to Text File(file (use dialog)=w342, text=w337, error in=w341) -> (refnum out=w345:refnum<file>, error out=w344:errorcluster)  [unwired: 1 in, 1 out]
            }
            n167 = Close File(refnum=w290, error in=w289) -> ()  [unwired: 2 out]
          }
        }
      }
      event "Analizza Dati": Value Change {
        n168 = event-data() -> ("NewVal"=w412:bool)  [unwired: 1 in, 5 out]
        n169 = case shown="True" w412 {
          tunnel: [w414 w420] -> w411
          tunnel: w410 -> [w414 w420]
          tunnel: [w415 w435] -> w409
          tunnel: w408 -> [w415 w435]
          tunnel: w407 -> [w416 w434]
          tunnel: [w416 w434] -> w406
          tunnel: [w413 w417] -> w402
          tunnel: w401 -> [w413 w417]
          frame False {
          }
          frame True {
            w433 = T3 0 items=["Least Square", "Least Absolute Residual", "Bisquare"] ("method")
            # "permette di graficare un polinomio su un certo range di valori\n(impostati come min e max valore dei miei valori letti da DAQ)"
            # "creazione linea fit"
            # "Cicolo for per crearmi i due array per le coordinate\ndei punti da mostrare nel grafico"
            # "Y array"
            # "X array"
            n170 = Array Size(array=w420) -> (size(s)=w421:i32[])
            n171 = Index Array(array=w421, index=1) -> (element=w422:i32)
            n172 = for {
              N: w422 -> [_]
              tunnel: w420 -> [w448]
              tunnel: [w442] -> w427 mode=indexing if=w436
              tunnel: [w441] -> w432 mode=indexing if=w436
              i -> [w445]
              n173 = Index Array(array=w448, index (row)=0, index (col)=w445) -> (element=w444:string)
              n174 = Index Array(array=w448, index (row)=1, index (col)=w445) -> (element=w443:string)
              n175 = Empty String/Path?(string/path=w443) -> (empty?=w439:bool)
              n176 = Empty String/Path?(string/path=w444) -> (empty?=w440:bool)
              n177 = Not(x=w439) -> (.not. x?=w438:bool)
              n178 = Fract/Exp String To Number(string=w444) -> (number=w442:dbl)  [unwired: 3 in, 1 out]
              n179 = Fract/Exp String To Number(string=w443) -> (number=w441:dbl)  [unwired: 3 in, 1 out]
              n180 = Not(x=w440) -> (.not. x?=w437:bool)
              n181 = And(x=w437, y=w438) -> (x .and. y?=w436:bool)
            }
            n182 = call <vilib>:"General Polynomial Fit.vi"("Y"=w432, "polynomial order"=w417, "X"=w427, "method"=w433) -> ("Polynomial Coefficients"=w430:dbl[])  [unwired: 8 in, 3 out]
            n183 = Bundle(w427, w432) -> (w426:cluster{dbl[], dbl[]})  [unwired: 1 in]
            n184 = Array Size(array=w427) -> (size(s)=w418:i32)
            n185 = Decrement(x=w418) -> (x-1=w419:i32)
            n186 = Index Array(array=w427, index=0) -> (element=w429:dbl)
            n187 = Index Array(array=w427, index=w419) -> (element=w428:dbl)
            n188 = call-poly <vilib>:"Polynomial Plot.vi"("P(x)"=w430, "end"=w428, "start"=w429) -> ("polynomial plot"=w425:cluster{"Ramp Pattern":dbl[], "P(A)":dbl[]})  [unwired: 7 in, 1 out]
            n189 = Build Array(w426, w425) -> (→"Graph":cluster{"Ramp Pattern":dbl[], "P(A)":dbl[]}[])
          }
        }
        n190 = property on="Analizza Dati" class="Bool (strict)"("Value"=FALSE ("Analizza Dati")) -> ()  [unwired: 2 in, 2 out]
      }
      event "Ordine Polinomio Fit": Value Change {
        n191 = event-data() -> ()  [unwired: 1 in, 6 out]
        n192 = property on="Analizza Dati" class="Bool (strict)"("Val(Sgnl)"=TRUE ("Value (Signaling)")) -> ()  [unwired: 2 in, 2 out]
        n193 = property on="Ordine Polinomio Fit" class="DigNum (strict)"() -> ("Value"=w449:i32)  [unwired: 2 in, 2 out]
      }
      event "stop": Value Change {
        # "Chiudere VI?"
        n194 = event-data() -> ()  [unwired: 1 in, 6 out]
      }
    }
    "Array" <- w26
  }
  n195 = property on="Tabella Acquisizioni" class="MCListbox (strict)"("AutoRowHt"=TRUE ("Autosizing Row Height"), "NumRows"=u32 2 ("Number of Rows")) -> ()  [unwired: 2 in, 2 out]
  n196 = property on="Stato Sensori" class="MCListbox (strict)"("ColHdrString"=string[] ["Indice", "Ingresso", "Sensore", "Descrizione", "AI min", "AI max", "Range", "Offset", "UM", "Funzione correttrice", "Ordine polinomio"] ("Row Header Strings[]")) -> ()  [unwired: 2 in, 2 out]
  n197 = property on="Graph" class="XYGraph (strict)"("Val(Sgnl)"=cluster{"Ramp Pattern":dbl[], "P(A)":dbl[]}[] [] ("Value (Signaling)")) -> ()  [unwired: 2 in, 2 out]
  n198 = property on="Ingresso Selezionato" class="Str"("Value"="" ("Sensore Selezionato")) -> ()  [unwired: 2 in, 2 out]
  n199 = property on="Analizza Dati" class="Bool (strict)"("Visible"=FALSE) -> ()  [unwired: 2 in, 2 out]
